vi "stopBaslerCamera.vi"   [LabVIEW 2012]
uses:
  GlobalBaslerCamera.vi
  <vilib>/vision/driver/NI_Vision_Acquisition_Software.lvlib
types:
  T1 = typedef "IMAQdx.ctl" = refnum<k21>
  T2 = typedef "IMAQ Image.ctl" = refnum<image>
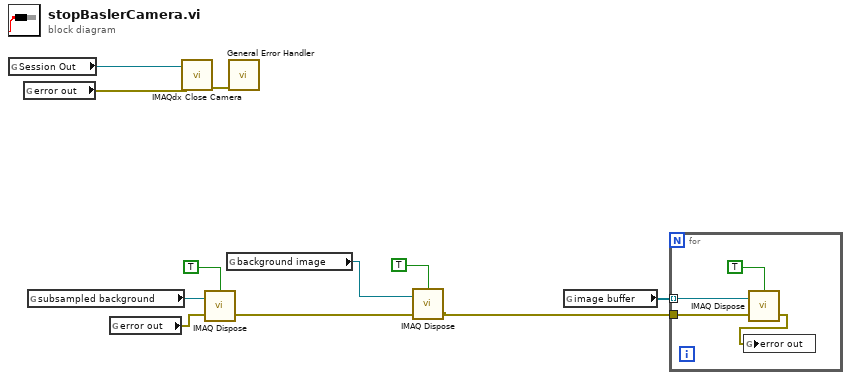
[diagram p0: block diagram]
diagram:
  n1 = global read "GlobalBaslerCamera.vi" "Session Out"() -> (w10:T1)
  n2 = global read "GlobalBaslerCamera.vi" "error out"() -> (w9:errorcluster)
  n3 = global read "GlobalBaslerCamera.vi" "subsampled background"() -> (w6:T2)
  n4 = global read "GlobalBaslerCamera.vi" "error out"() -> (w2:errorcluster)
  n5 = call <vilib>:"IMAQdx Close Camera.vi"("error in"=w9, "Session In"=w10) -> ("error out"=w11:errorcluster)  [unwired: 9 out]
  n6 = call "IMAQ Dispose"("All Images? (No)"=TRUE, "Image"=w6, "error in (no error)"=w2) -> ("error out"=w3:errorcluster)  [unwired: 3 in]
  n7 = global read "GlobalBaslerCamera.vi" "background image"() -> (w4:T2)
  n8 = call <vilib>:"General Error Handler.vi"("error in (no error)"=w11) -> ()  [unwired: 1 in, 14 out]
  n9 = call "IMAQ Dispose"("All Images? (No)"=TRUE, "Image"=w4, "error in (no error)"=w3) -> ("error out"=w1:errorcluster)  [unwired: 3 in]
  n10 = global read "GlobalBaslerCamera.vi" "image buffer"() -> (w8:T2[])
  n11 = for {
    tunnel: w8 -> [w15] mode=indexing
    tunnel: w1 -> [w13]
    n12 = call "IMAQ Dispose"("All Images? (No)"=TRUE, "Image"=w15, "error in (no error)"=w13) -> ("error out"=w12:errorcluster)  [unwired: 3 in]
    n13 = global write "GlobalBaslerCamera.vi" "error out"(w12) -> ()
  }
